vi "GateSTS.vi"(5 "Store\nSecond Gate?":bool, 6 "Attributes":string[][](array[string]), 10 "Basename":string) -> (3 "Stop Loop":bool)   [LabVIEW 2021]
uses:
  <userlib>/Nanonis Prog Interface V5/Nanonis Prog Interface.lvlib
panel:
  in  "Tabs":T1(tab)
  in  "Start Gate (V)":dbl
  in  "End Gate (V)":dbl
  in  "Increment Gate (V)":dbl
  in  "Stop":bool
  out "Current Gate Voltage (V)":dbl
  in  "?":bool
  out "HDF5 DATANAME":string
  in  "Store\nLock-in\nParameters?":bool=TRUE
  in  "Store\nTemperatures?":bool
  in  "Store\nMagnetic Field?":bool
  in  "Zigzag Raster?":bool
  in  "Insert Loop Index\ninto Basename?":bool
  in  "Loop Forever?":bool
  out "Loop Index":i32
  in  "Loop Index Offset":i32=1
  in  "Make .dat files?":bool
  out "Ender":bool
  # "Gate STS"
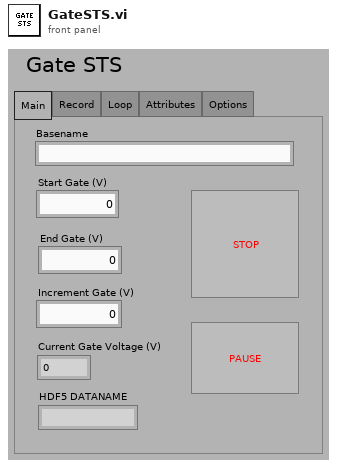
[diagram p1: front panel]
types:
  T1 = enum32{"Main", "Record", "Loop", "Attributes", "Options"}
  T2 = cluster{"Save all":enum16{"no change", "on", "off"}, "Number of Sweeps (0=no change)":i32}
  T3 = enum16{"Set Voltage", "Read Voltage", "Read Current", "Output On", "Output Off", "Set Increment", "Set Increment Time", "Stop Voltage Set", "Set Maximum Voltage", "Get Maximum Voltage"}
  T4 = enum16{"Output 2 (V)", "Output 3 (V)", "Output 4 (V)"}
  T5 = enum16{"Read State", "Hold", "Ramp to Set", "Ramp to Zero", "Read Switch Heater", "Switch Heater On", "Switch Heater Off", "Read Voltage", "Read Current", "Read Field", "Read Persistent Field", "Read Target Field", "Set Target Field", "Read Ramp Rate", "Set Ramp Rate"}
  T6 = enum16{"pot_temp", "sorb_temp", "needle_valve_temp", "still_temp", "mix_chamber_temp", "stm_rx_temp", "stm_cx_temp", "tank_pressure", "condense_pressure", "still_pressure", "turbo_back_pressure", "n2_trap_pressure"}
  T7 = enum16{"Set Amplitude", "Get Amplitude", "Set Frequency", "Get Frequency", "Set Harmonic", "Get Harmonic", "Set Phase", "Get Phase", "Auto Phase", "Add to Phase", "Autogain", "Set Time Constant", "Get Time Constant", "Set Sensitivity", "Get Sensitivity", "Set Input A", "Set Input A-B", "Get Input Setting", "Set Offset", "Get Offset"}[]
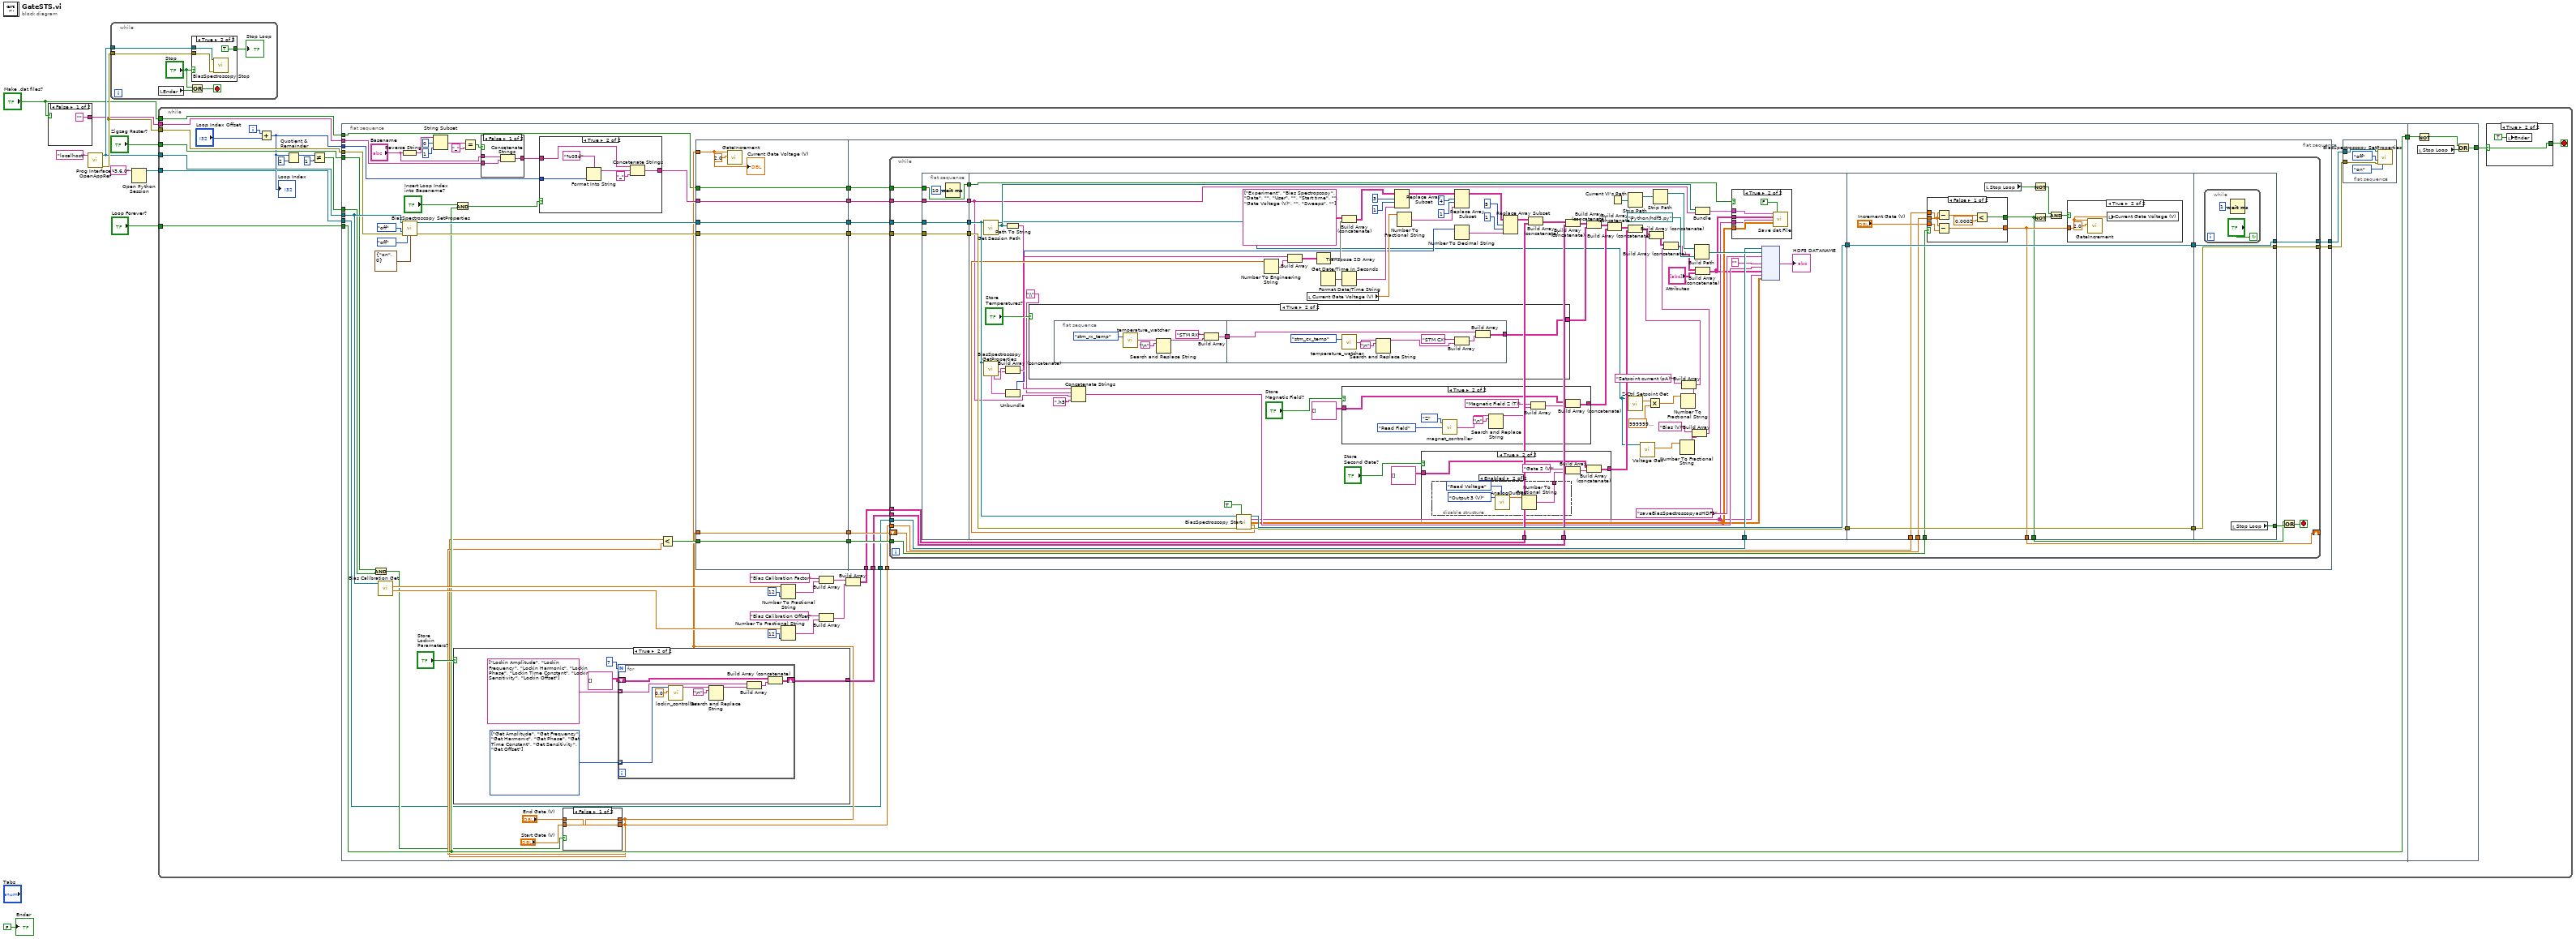
[diagram p0: block diagram]
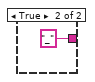
[diagram p2: hidden frame]
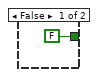
[diagram p3: hidden frame]
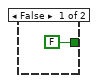
[diagram p4: hidden frame]
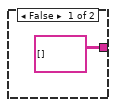
[diagram p8: hidden frame]
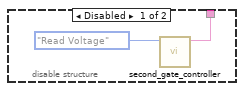
[diagram p10: hidden frame]
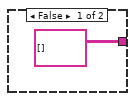
[diagram p13: hidden frame]
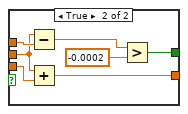
[diagram p14: hidden frame]
diagram:
  n1 = case shown="False" "Make .dat files?" {
    tunnel: ["" ("string") "_" ("string")] -> w2
    frame False {
    }
    frame True {
    }
  }
  n2 = call <userlib>:"Prog Interface - OpenAppRef.vi"("Machine name (local machine IP)"="localhost" ("machine name (localhost)")) -> ("Error out"=w7:errorcluster, "Application reference"=w6:refnum<vi>)  [unwired: 5 in]
  n3 = while {
    tunnel: w6 -> [w18]
    tunnel: w7 -> [w17]
    stop <- w14 stop-if-true
    n4 = local read "Ender"() -> (w13:bool)
    n5 = Or(x="Stop", y=w13) -> (x .or. y?=w14:bool)
    n6 = case shown="True" "Stop" {
      tunnel: w18 -> [_ w22]
      tunnel: w17 -> [_ w21]
      tunnel: [FALSE TRUE] -> w16
      frame False {
      }
      frame True {
        n7 = call <userlib>:"BiasSpectroscopy Stop.vi"("Application ref in"=w22, "Error in (no error)"=w21) -> ()  [unwired: 12 in, 2 out]
      }
    }
    "Stop Loop" <- w16
  }
  n8 = Open Python Session(python version="3.6.0" ("Python version")) -> (session out=w4:refnum<k35>)  [unwired: 2 in, 1 out]
  n9 = while {
    tunnel: "Loop Forever?" -> [w39]
    tunnel: w6 -> [w37]
    tunnel: w7 -> [w36]
    tunnel: "Zigzag Raster?" -> [w32]
    tunnel: w4 -> [w25]
    tunnel: w2 -> [w24]
    tunnel: "Make .dat files?" -> [w23]
    i -> [w33]
    stop <- w34 stop-if-true
    n10 = Add(x=w33, y="Loop Index Offset") -> (x+y=w30:i32)
    "Loop Index" <- w30
    n11 = Quotient & Remainder(x=w30, y=2) -> (x-y*floor(x/y)=w28:i32)  [unwired: 1 out]
    n12 = Not Equal?(x=w28, y=1) -> (x != y?=w26:bool)
    n13 = flat-sequence {
      tunnel: w39 -> [w64]
      tunnel: [w64] -> w38
      tunnel: w37 -> [w68]
      tunnel: w36 -> [w67]
      tunnel: w30 -> [w62]
      tunnel: w32 -> [w49]
      tunnel: w26 -> [w48]
      tunnel: w25 -> [w46]
      tunnel: w24 -> [w45]
      tunnel: w23 -> [w43]
      tunnel: w38 -> [w337]
      tunnel: [w334] -> w35
      frame #0 {
        n14 = And(x=w49, y=w48) -> (x .and. y?=w47:bool)
        n15 = call <userlib>:"Bias Calibration Get.vi"("Application ref in"=w68) -> ("Offset (V)"=w78:sgl, "Calibration (V/V)"=w79:sgl)  [unwired: 7 in, 2 out]
        n16 = Reverse String(1:"Basename") -> (0:w59:string)
        n17 = call <userlib>:"BiasSpectroscopy SetProperties.vi"("Application ref in"=w68, "Autosave (no change)"=enum16{"no change", "on", "off"}."off", "Error in (no error)"=w67, "Save dialog"=enum16{"no change", "on", "off"}."off", "Multiple sweeps config"=T2 {"Save all"=enum."on", "Number of Sweeps (0=no change)"=0}) -> ("Application ref out"=w88:refnum<vi>, "Error out"=w89:errorcluster)  [unwired: 9 in]
        n18 = String Subset(string=w59, offset (0)=0, length (rest)=1 ("length (rest)")) -> (substring=w58:string)
        n19 = case shown="True" "Store\nLock-in\nParameters?" {
          tunnel: [string[][] [] w111] -> w80
          frame False {
          }
          frame True {
            w114 = T7 [enum."Get Amplitude", enum."Get Frequency", enum."Get Harmonic", enum."Get Phase", enum."Get Time Constant", enum."Get Sensitivity", enum."Get Offset"] items=["Set Amplitude", "Get Amplitude", "Set Frequency", "Get Frequency", "Set Harmonic", "Get Harmonic", "Set Phase", "Get Phase", "Auto Phase", "Add to Phase", "Autogain", "Set Time Constant", "Get Time Constant", "Set Sensitivity", "Get Sensitivity", "Set Input A", "Set Input A-B", "Get Input Setting", "Set Offset", "Get Offset"]
            n20 = for {
              N: 7 -> [_]
              tunnel: w114 -> [w122] mode=indexing
              tunnel: string[] ["Lockin Amplitude", "Lockin Frequency", "Lockin Harmonic", "Lockin Phase", "Lockin Time Constant", "Lockin Sensitivity", "Lockin Offset"] -> [w121] mode=indexing
              shift-right: [w119] -> w111
              shift-left: string[][] [] -> [w120]
              n21 = call "lockin_controller.vi"("Numerical Argument"=0.0, "Command"=w122) -> ("Response"=w117:string)  [unwired: 9 in]
              n22 = Search and Replace String(input string=w117, search string="\n") -> (result string=w118:string)  [unwired: 6 in, 3 out]
              n23 = Build Array(w121, w118) -> (w123:string[])
              n24 = Build Array (concatenate)(w120, w123) -> (w119:string[][])
            }
          }
        }
        n25 = And(x="Insert Loop Index\ninto Basename?", y=w64) -> (x .and. y?=w63:bool)
        n26 = Equal?(x=w58, y="_") -> (x = y?=w56:bool)
        n27 = case shown="False" w56 {
          tunnel: "Basename" -> [w101 w102]
          tunnel: [w100 w102] -> w54
          tunnel: w45 -> [w99 _]
          frame False {
            n28 = Concatenate Strings(w101, w99) -> (w100:string)
          }
          frame True {
          }
        }
        n29 = case shown="True" w63 {
          tunnel: [w103 w109] -> w66
          tunnel: w54 -> [w103 w108]
          tunnel: w62 -> [_ w106]
          frame False {
          }
          frame True {
            n30 = Format Into String(format string="%05d", w106) -> (resulting string=w104:string)  [unwired: 2 in, 1 out]
            n31 = Concatenate Strings(w108, w104, "_" ("string")) -> (w109:string)
          }
        }
        n32 = case shown="False" w47 {
          tunnel: "End Gate (V)" -> [w96 w98]
          tunnel: [w96 w97] -> w52
          tunnel: [w95 w98] -> w51
          tunnel: "Start Gate (V)" -> [w95 w97]
          frame False {
          }
          frame True {
          }
        }
        n33 = Less?(x=w51, y=w52) -> (x < y?=w83:bool)
        n34 = flat-sequence {
          tunnel: w51 -> [w132]
          tunnel: w83 -> [w133]
          tunnel: w88 -> [w134]
          tunnel: w89 -> [w135]
          tunnel: w66 -> [w136]
          tunnel: [w136] -> w94
          tunnel: [w135] -> w93
          tunnel: [w134] -> w92
          tunnel: [w133] -> w91
          tunnel: [w132] -> w90
          tunnel: w51 -> [w130]
          tunnel: [w129] -> w44
          tunnel: w43 -> [w129]
          tunnel: [w145] -> w86
          tunnel: [w144] -> w85
          tunnel: w94 -> [w148]
          tunnel: w93 -> [w147]
          tunnel: w92 -> [w146]
          tunnel: w91 -> [w143]
          tunnel: w90 -> [w142]
          tunnel: w52 -> [w141]
          tunnel: w80 -> [w140]
          tunnel: w69 -> [w139]
          tunnel: w46 -> [w138]
          tunnel: w44 -> [w137]
          frame #0 {
            n35 = call "GateIncrement.vi"("Increment"=2.0, "Gate Voltage"=w130) -> ()  [unwired: 10 in]
            "Current Gate Voltage (V)" <- w130
          }
          frame #1 {
            n36 = while {
              tunnel: w148 -> [w172]
              tunnel: w147 -> [w171]
              tunnel: w146 -> [w170]
              tunnel: [w169] -> w145
              tunnel: [w168] -> w144
              tunnel: w143 -> [w154]
              shift-right: [w158] -> _
              shift-left: w142 -> [w156]
              tunnel: w141 -> [w155]
              tunnel: w140 -> [w153]
              tunnel: w139 -> [w152]
              tunnel: w138 -> [w151]
              tunnel: w137 -> [w149]
              stop <- w159 stop-if-true
              n37 = flat-sequence {
                tunnel: w170 -> [w175]
                tunnel: w171 -> [w176]
                tunnel: w172 -> [w177]
                tunnel: [w177] -> w163
                tunnel: [w176] -> w162
                tunnel: [w175] -> w161
                tunnel: [w173] -> w150
                tunnel: w149 -> [w173]
                tunnel: [w254] -> w165
                tunnel: [w255] -> w164
                tunnel: w163 -> [w211]
                tunnel: w162 -> [w256]
                tunnel: w161 -> [w252]
                tunnel: w153 -> [w227]
                tunnel: w152 -> [w225]
                tunnel: w151 -> [w214]
                tunnel: w150 -> [w200]
                tunnel: [w312] -> w167
                tunnel: [w311] -> w166
                tunnel: w165 -> [w312]
                tunnel: w164 -> [w311]
                tunnel: [w307] -> w158
                tunnel: [w305] -> w157
                tunnel: w156 -> [w304]
                tunnel: w155 -> [w302]
                tunnel: w154 -> [w301]
                tunnel: [w330] -> w169
                tunnel: [w331] -> w168
                tunnel: w167 -> [w331]
                tunnel: w166 -> [w330]
                tunnel: [w329] -> w160
                frame #0 {
                  n38 = Wait (ms)(milliseconds to wait=u32 10) -> ()  [unwired: 1 out]
                }
                frame #1 {
                  n39 = call <userlib>:"Get Session Path.vi"("Application ref in"=w252) -> ("Session path"=w212:path, "Application ref out"=w184:refnum<vi>)  [unwired: 8 in, 1 out]
                  n40 = call <userlib>:"BiasSpectroscopy GetProperties.vi"("Application ref in"=w252) -> ("Parameters"=w244:string[], "Multiple sweeps configuration"=w233:cluster{"Number of Sweeps":i32, "Save all":bool}, "Fixed parameters"=w245:string[])  [unwired: 7 in, 5 out]
                  n41 = Unbundle(w233) -> ("Number of Sweeps"=w232:i32)  [unwired: 1 out]
                  n42 = Path To String(path=w212) -> (string=w205:string)
                  n43 = Build Array (concatenate)(w245, w244) -> (w249:string[])
                  n44 = case shown="True" "Store\nTemperatures?" {
                    tunnel: [string[][] [] w285] -> w221
                    frame False {
                    }
                    frame True {
                      n45 = flat-sequence {
                        tunnel: [w290] -> w286
                        tunnel: w286 -> [w297]
                        tunnel: [w296] -> w285
                        frame #0 {
                          n46 = call "temperature_watcher.vi"("Command"=T6."stm_rx_temp") -> ("Response"=w288:string)  [unwired: 1 in]
                          n47 = Search and Replace String(input string=w288, search string="\n") -> (result string=w287:string)  [unwired: 6 in, 3 out]
                          n48 = Build Array("STM RX" ("element"), w287) -> (w290:string[])
                        }
                        frame #1 {
                          n49 = call "temperature_watcher.vi"("Command"=T6."stm_cx_temp") -> ("Response"=w294:string)  [unwired: 1 in]
                          n50 = Search and Replace String(input string=w294, search string="\n") -> (result string=w293:string)  [unwired: 6 in, 3 out]
                          n51 = Build Array("STM CX" ("element"), w293) -> (w298:string[])
                          n52 = Build Array(w297, w298) -> (w296:string[][])
                        }
                      }
                    }
                  }
                  n53 = Concatenate Strings(w205, "\\" ("string"), w211, ".h5" ("string")) -> (w209:string)
                  n54 = call <userlib>:"BiasSpectroscopy Start.vi"("Application ref in"=w252, "Get data (F)"=TRUE, "Error in (no error)"=w256) -> ("Application ref out"=w255:refnum<vi>, "Channels"=w202:string[], "Data"=w203:sgl[][], "Parameters"=w251:sgl[], "Error out"=w254:errorcluster)  [unwired: 8 in]
                  n55 = Number To Engineering String(4:w251) -> (0:w250:string[])  [unwired: 3 in]
                  n56 = Build Array(w249, w250) -> (w248:string[][])
                  n57 = local read "Current Gate Voltage (V)"() -> (w235:dbl)
                  n58 = Transpose 2D Array(2D array=w248) -> (transposed array=w246:string[][])
                  n59 = Get Date/Time In Seconds() -> (seconds since 1Jan1904=w243:timestamp)
                  n60 = Build Array (concatenate)(string[][] [["Experiment", "Bias Spectroscopy"], ["Date", ""], ["User", ""], ["Start time", ""], ["Gate Voltage (V)", ""], ["Sweeps", ""]] ("Attributes"), w246) -> (w242:string[][])
                  n61 = Format Date/Time String(seconds (now)=w243) -> (date/time string=w241:string)  [unwired: 2 in]
                  n62 = case shown="True" "Store\nMagnetic Field?" {
                    tunnel: [w274 w278] -> w218
                    tunnel: string[][] [] ("array") -> [w274 w279]
                    frame False {
                    }
                    frame True {
                      n63 = call "magnet_controller.vi"("Command"=T5."Read Field", "Direction"=enum16{"X", "Y", "Z"}."Z") -> ("Response"=w276:string)  [unwired: 1 in]
                      n64 = Search and Replace String(input string=w276, search string="\n") -> (result string=w275:string)  [unwired: 6 in, 3 out]
                      n65 = Build Array("Magnetic Field Z (T)" ("element"), w275) -> (w280:string[])
                      n66 = Build Array (concatenate)(w279, w280) -> (w278:string[][])
                    }
                  }
                  n67 = Replace Array Subset(array=w242, new element=w241, index (row)=3, index (col)=1 ("disabled index (col)")) -> (w238:string[][])
                  n68 = Number To Fractional String(number=w235) -> (F-format string=w234:string)  [unwired: 3 in]
                  n69 = case shown="True" "Store\nSecond Gate?" {
                    tunnel: [w257 w259] -> w192
                    tunnel: string[][] [] ("array") -> [w257 w260]
                    frame False {
                    }
                    frame True {
                      n70 = disable-structure shown="Enabled" {
                        disable-tunnel: [w264 w268] -> w258
                        frame Disabled {
                          n71 = call "second_gate_controller.vi"("Command"=T3."Read Voltage") -> ("Response"=w264:string)  [unwired: 10 in]
                        }
                        frame Enabled {
                          n72 = call "AnalogOutput.vi"("Read or Set Voltage?"=enum16{"Read Voltage", "Set Voltage"}."Read Voltage", "Channel"=T4."Output 3 (V)") -> ("Output Voltage"=w267:sgl)  [unwired: 9 in]
                          n73 = Number To Fractional String(number=w267) -> (F-format string=w268:string)  [unwired: 3 in]
                        }
                      }
                      n74 = Build Array("Gate 2 (V)" ("element"), w258) -> (w261:string[])
                      n75 = Build Array (concatenate)(w260, w261) -> (w259:string[][])
                    }
                  }
                  n76 = Replace Array Subset(array=w238, new element=w234, index (row)=4, index (col)=1 ("disabled index (col)")) -> (w231:string[][])
                  n77 = Number To Decimal String(number=w232) -> (decimal integer string=w228:string)  [unwired: 1 in]
                  n78 = Replace Array Subset(array=w231, new element=w228, index (row)=5, index (col)=1 ("disabled index (col)")) -> (w226:string[][])
                  n79 = Build Array (concatenate)(w226, w225) -> (w224:string[][])
                  n80 = Build Array (concatenate)(w224, w227) -> (w222:string[][])
                  n81 = Build Array (concatenate)(w222, w221) -> (w219:string[][])
                  n82 = Build Array (concatenate)(w219, w218) -> (w195:string[][])
                  n83 = Current VI's Path() -> (path=w206:path)
                  n84 = Strip Path(path=w206) -> (stripped path=w207:path)  [unwired: 1 out]
                  n85 = Build Array (concatenate)(w195, w192) -> (w191:string[][])
                  n86 = call <userlib>:"Z-Ctrl Setpoint Get.vi"("Application ref in"=w184) -> ("Z Controller setpoint"=w180:sgl)  [unwired: 7 in, 2 out]
                  n87 = call <userlib>:"Voltage Get.vi"("Application ref in"=w184) -> ("Bias (V)"=w185:sgl)  [unwired: 8 in, 2 out]
                  n88 = Multiply(x=w180, y=sgl 1000000000000.0) -> (x*y=w178:sgl)
                  n89 = Strip Path(path=w207) -> (stripped path=w208:path)  [unwired: 1 out]
                  n90 = Number To Fractional String(number=w185) -> (F-format string=w187:string)  [unwired: 3 in]
                  n91 = Number To Fractional String(number=w178) -> (F-format string=w190:string)  [unwired: 3 in]
                  n92 = Build Array("Setpoint current (pA)" ("element"), w190) -> (w188:string[])
                  n93 = Build Array (concatenate)(w191, w188) -> (w183:string[][])
                  n94 = Build Array("Bias (V)" ("element"), w187) -> (w182:string[])
                  n95 = Build Array (concatenate)(w183, w182) -> (w181:string[][])
                  n96 = Build Path(base path=w208, name or relative path=path "Python/hdf5.py") -> (appended path=w215:path)
                  n97 = Bundle("Session path"=w212, "Basename"=w211) -> (w201:cluster{"Session path":path, "Basename":string})  [unwired: 1 in]
                  n98 = Build Array (concatenate)(w181, "Attributes") -> (w196:string[][])
                  n99 = case shown="True" w200 {
                    tunnel: w196 -> [_ w273]
                    tunnel: w203 -> [_ w272]
                    tunnel: w202 -> [_ w271]
                    tunnel: w201 -> [_ w270]
                    frame False {
                    }
                    frame True {
                      n100 = call <userlib>:"Save dat File.vi"("Filename control"=w270, "Show save dialog (T)"=FALSE, "Attributes"=w273, "Channels names"=w271, "Data"=w272) -> ()  [unwired: 7 in, 4 out]
                    }
                  }
                  n101 = node(w214, w215, "saveBiasSpectroscopyasHDF5" ("function name"), "" ("function name"), w209, w196, w202, w203) -> (→"HDF5 DATANAME":string)  [unwired: 5 in, 4 out]
                }
                frame #2 {
                  n102 = case shown="False" w301 {
                    tunnel: w304 -> [w317 w323]
                    tunnel: "Increment Gate (V)" -> [w318 w326]
                    tunnel: [w319 w325] -> w307
                    tunnel: w302 -> [w316 w324]
                    tunnel: [w314 w322] -> w305
                    frame False {
                      n103 = Subtract(x=w317, y=w316) -> (x-y=w315:dbl)
                      n104 = Subtract(x=w317, y=w318) -> (x-y=w319:dbl)
                      n105 = Less?(x=w315, y=0.0002) -> (x < y?=w314:bool)
                    }
                    frame True {
                      n106 = Subtract(x=w323, y=w324) -> (x-y=w321:dbl)
                      n107 = Add(x=w323, y=w326) -> (x+y=w325:dbl)
                      n108 = Greater?(x=w321, y=-0.0002) -> (0:w322:bool)
                    }
                  }
                  n109 = local read "Stop Loop"() -> (w310:bool)
                  n110 = Not(x=w310) -> (.not. x?=w308:bool)
                  n111 = Not(x=w305) -> (.not. x?=w306:bool)
                  n112 = And(x=w308, y=w306) -> (x .and. y?=w309:bool)
                  n113 = case shown="True" w309 {
                    tunnel: w307 -> [_ w328]
                    frame False {
                    }
                    frame True {
                      n114 = call "GateIncrement.vi"("Increment"=2.0, "Gate Voltage"=w328) -> ()  [unwired: 10 in]
                      n115 = local write "Current Gate Voltage (V)"(w328) -> ()
                    }
                  }
                }
                frame #3 {
                  n116 = while {
                    stop <- "?" continue-if-true
                    n117 = Wait (ms)(milliseconds to wait=u32 1) -> ()  [unwired: 1 out]
                  }
                  n118 = local read "Stop Loop"() -> (w329:bool)
                }
              }
              n119 = Or(x=w157, y=w160) -> (x .or. y?=w159:bool)
            }
          }
        }
        n120 = Number To Fractional String(number=w79, precision (6)=i16 12) -> (F-format string=w75:string)  [unwired: 2 in]
        n121 = Number To Fractional String(number=w78, precision (6)=i16 12) -> (F-format string=w72:string)  [unwired: 2 in]
        n122 = Build Array("Bias Calibration Factor" ("element"), w75) -> (w70:string[])
        n123 = Build Array("Bias Calibration Offset" ("element"), w72) -> (w71:string[])
        n124 = Build Array(w70, w71) -> (w69:string[][])
        n125 = flat-sequence {
          tunnel: w86 -> [w128]
          tunnel: w85 -> [w127]
          frame #0 {
            n126 = call <userlib>:"BiasSpectroscopy SetProperties.vi"("Application ref in"=w128, "Autosave (no change)"=enum16{"no change", "on", "off"}."off", "Error in (no error)"=w127, "Save dialog"=enum16{"no change", "on", "off"}."on") -> ()  [unwired: 10 in, 2 out]
          }
        }
      }
      frame #1 {
        n127 = Not(x=w337) -> (.not. x?=w335:bool)
        n128 = local read "Stop Loop"() -> (w336:bool)
        n129 = Or(x=w335, y=w336) -> (x .or. y?=w334:bool)
      }
    }
    n130 = case shown="True" w35 {
      selector: w35 -> [_ w42]
      tunnel: [FALSE w42] -> w34
      frame False {
      }
      frame True {
        n131 = local write "Ender"(TRUE ("Ender")) -> ()
      }
    }
  }
  "Ender" <- FALSE ("Ender")
